vi "Arm2Global.vi"() -> ()   [LabVIEW 2023]
doc: "Arm global (getters and setter stuff)"
panel:
  out "Arm2Position(Degrees)":dbl
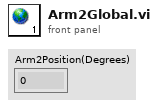
[diagram p1: front panel]
diagram:
